vi "Values String Changed.vi"(8 "error in (no error)":errorcluster, 11 "Application Data in":T1 {"current buffer data"."channels"."configuration"."string offset" format="%d bytes"; "current buffer data"."avg bandwidth" format="%.0g bytes"}) -> (0 "error out":errorcluster, 3 "Application Data out":T1 {"current buffer data"."channels"."configuration"."string offset" format="%d bytes"; "current buffer data"."avg bandwidth" format="%.0g bytes"})   [LabVIEW 2017, in "Data Viewer.lvlib"]
uses:
  Core/VIs/Data Viewer/Source/Data Viewer.lvlib
  Application Data.ctl
  <vilib>/NI/Memory Manager/Classes/Pointer/Pointer.lvclass
  VeriStand/Data Sharing Custom Device/Source/DSF Core.lvlibp/Classes/Configuration/Core/Framework/Framework Configuration.lvclass
  Buffer Reader/Queue Data.ctl
  Buffer Reader/Buffer Data.ctl
  VeriStand/Data Sharing Custom Device/Source/DSF Core.lvlibp/Classes/Configuration/Core/Transfer/Channel Configuration.ctl
  VeriStand/Data Sharing Custom Device/Source/DSF Core.lvlibp/Typedefs/Core Channel Configuration.ctl
  VeriStand/Data Sharing Custom Device/Source/DSF Core.lvlibp/Typedefs/DSF Data Type.ctl
  VeriStand/Data Sharing Custom Device/Source/DSF Core.lvlibp/Typedefs/DSF Settings Info.ctl
  VeriStand/Data Sharing Custom Device/Source/DSF Core.lvlibp/Typedefs/DSF Byte Order.ctl
  VeriStand/Data Sharing Custom Device/Source/DSF Core.lvlibp/Classes/Thread/Data Server/DSF Buffer Subset Descriptor.ctl
  VeriStand/Data Sharing Custom Device/Source/DSF Core.lvlibp/Typedefs/DSF Buffer Type.ctl
  Values Channels.ctl
  VeriStand/Data Sharing Custom Device/Source/DSF Core.lvlibp/Classes/Framework/Framework.lvclass
  VeriStand/Data Sharing Custom Device/Source/DSF Core.lvlibp
  VeriStand/Data Sharing Custom Device/Source/DSF Core.lvlibp/Classes/Configuration/Core/Channel/Channel Configuration.lvclass
  VeriStand/Data Sharing Custom Device/Source/DSF Core.lvlibp/Classes/Configuration/Core/Transfer/Transfer Configuration.lvclass
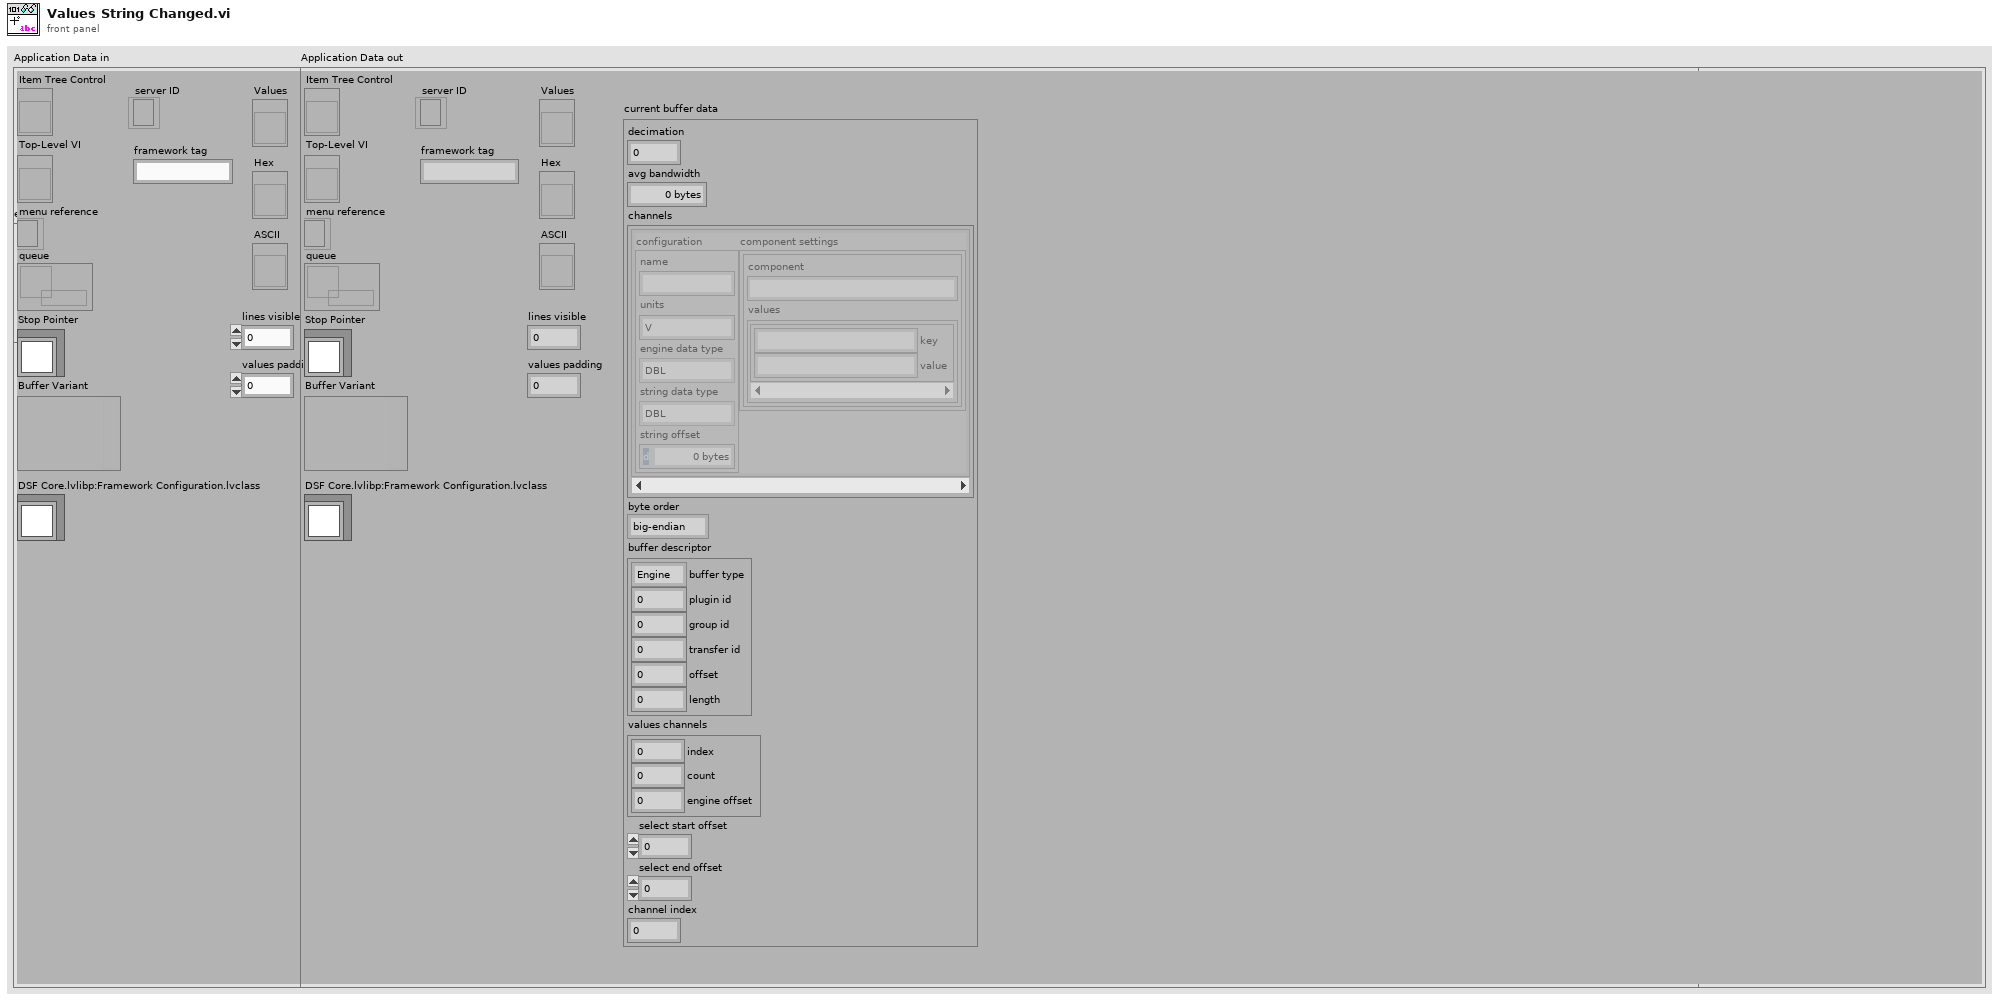
[diagram p1: front panel]
types:
  T1 = typedef "Data Viewer.lvlib/Application Data.ctl" = cluster{"Item Tree Control":refnum<vi>, "Top-Level VI":refnum<vi>, "menu reference":refnum<k9>, "queue":refnum<queue>, "Stop Pointer":refnum<class "Pointer.lvclass">, "Buffer Variant":variant, "server ID":refnum<k5>, "framework tag":string, "Values":refnum<vi>, "Hex":refnum<vi>, "ASCII":refnum<vi>, "lines visible":i32, "values padding":i32, "current buffer data":T2, "DSF Core.lvlibp:Framework Configuration.lvclass":refnum<class "Framework Configuration.lvclass">}
  T2 = typedef "Data Viewer.lvlib/Buffer Data.ctl" = cluster{"decimation":u64, "avg bandwidth":dbl, "channels":T3[], "byte order":T7, "buffer descriptor":T8, "values channels":T10, "select start offset":u64, "select end offset":u64, "channel index":i32}
  T3 = typedef "DSF Core.lvlibp/Transfer Configuration.lvclass/Channel Configuration.ctl" = cluster{"configuration":T4, "component settings":T6[]}
  T4 = typedef "DSF Core.lvlibp/Channel Configuration.lvclass/Core Channel Configuration.ctl" = cluster{"name":string, "units":string, "engine data type":T5, "string data type":T5, "string offset":u64}
  T5 = typedef "DSF Core.lvlibp/DSF Data Type.ctl" = enum8{"Bool", "SGL", "DBL", "I8", "I16", "I32", "I64", "U8", "U16", "U32", "U64"}
  T6 = typedef "DSF Core.lvlibp/DSF Settings Info.ctl" = cluster{"component":string, "values":cluster{"key":string, "value":string}[]}
  T7 = typedef "DSF Core.lvlibp/DSF Byte Order.ctl" = enum8{"big-endian", "little-endian"}
  T8 = typedef "DSF Core.lvlibp/DSF Buffer Subset Descriptor.ctl" = cluster{"buffer type":T9, "plugin id":i32, "group id":i32, "transfer id":i32, "offset":u64, "length":i64}
  T9 = typedef "DSF Core.lvlibp/DSF Buffer Type.ctl" = enum16{"Engine", "String"}
  T10 = typedef "Data Viewer.lvlib/Values Channels.ctl" = cluster{"index":i32, "count":i32, "engine offset":u64}
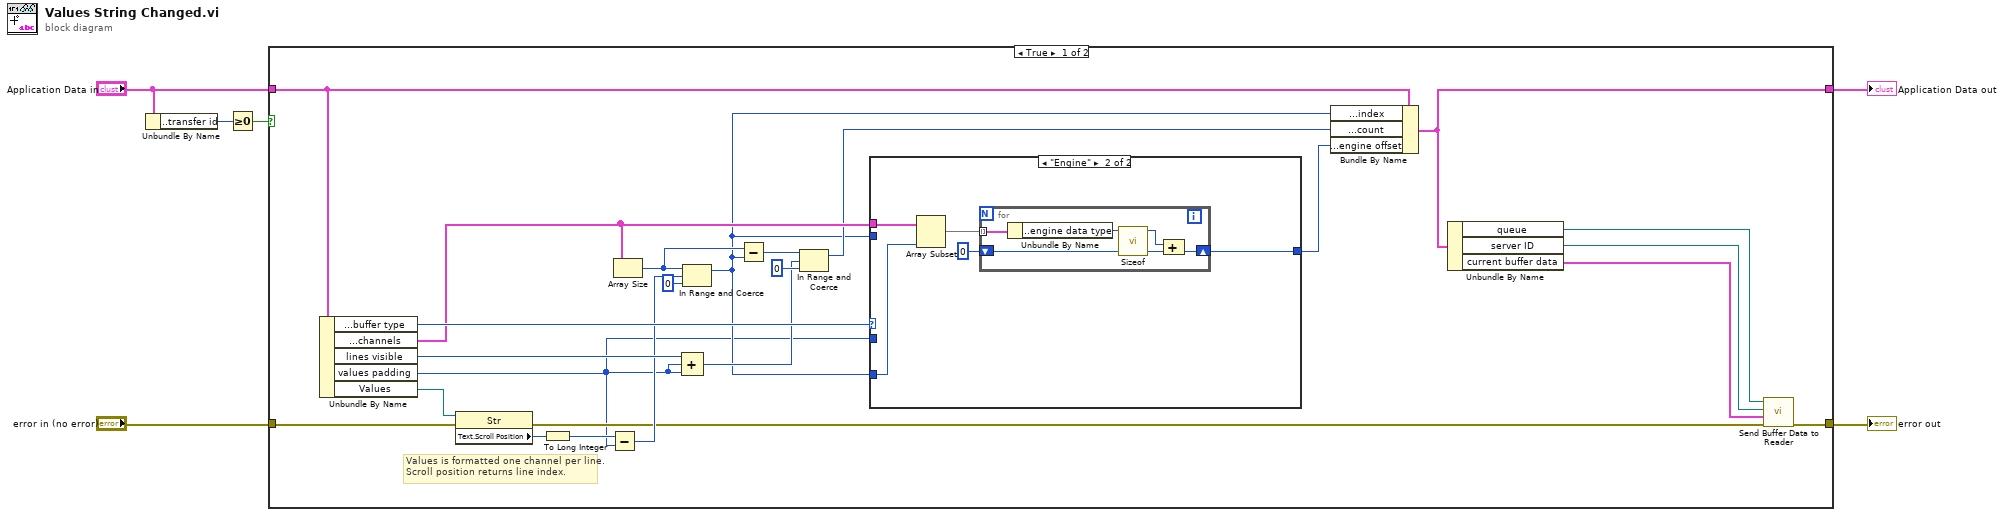
[diagram p0: block diagram]
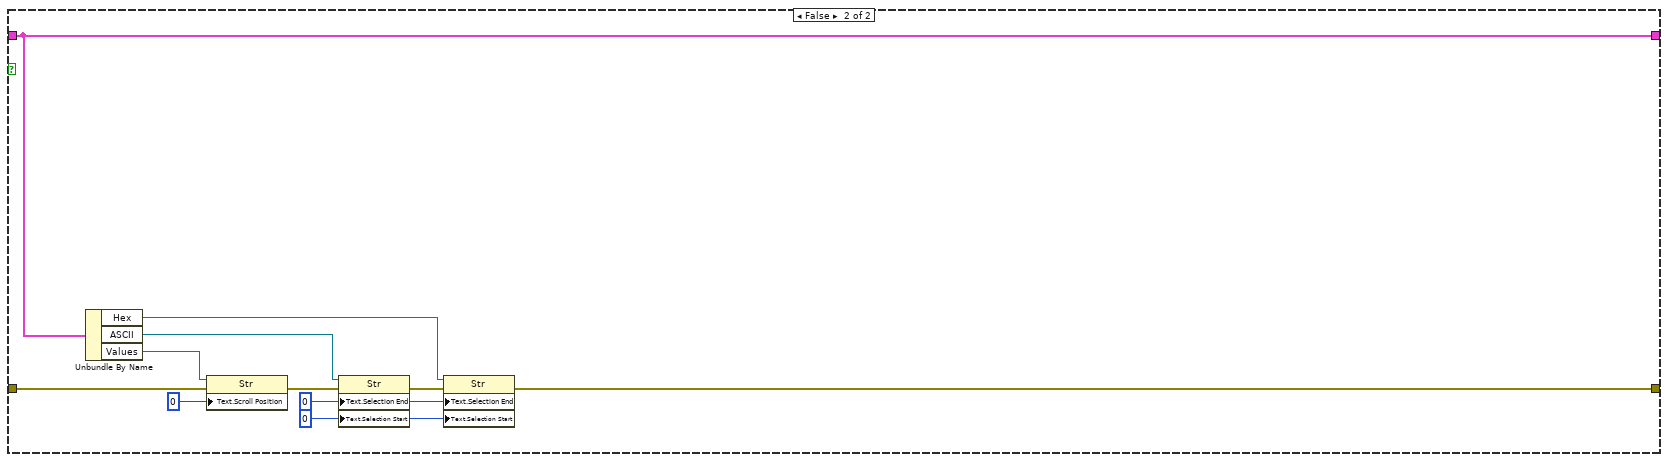
[diagram p3: hidden frame]
diagram:
  n1 = Unbundle By Name("Application Data in") -> ("current buffer data.buffer descriptor.transfer id"=w1:i32)
  n2 = Greater Or Equal To 0?(x=w1) -> (x >= 0?=w2:bool)
  n3 = case shown="True" w2 {
    tunnel: "error in (no error)" -> [w30 w50]
    tunnel: [w22 w47] -> w4
    tunnel: "Application Data in" -> [w25 w49]
    tunnel: [w18 w49] -> w5
    frame True {
      # "Values is formatted one channel per line. Scroll position returns line index."
      n4 = Unbundle By Name(w25) -> ("current buffer data.buffer descriptor.buffer type"=w24:T9, "current buffer data.channels"=w23:T3[], "lines visible"=w16:i32, "values padding"=w7:i32, "Values"=w26:refnum<vi>)
      n5 = property class="Str"(reference=w26, error in=w30) -> (error out=w8:errorcluster, "Text.Scroll Position"=w28:u32)  [unwired: 1 out]
      n6 = To Long Integer(number=w28) -> (32bit integer=w27:i32)
      n7 = Subtract(x=w27, y=w7) -> (x-y=w15:i32)
      n8 = Array Size(array=w23) -> (size(s)=w14:i32)
      n9 = Compound Arithmetic op=ADD(w16, w7, w7) -> (w10:i32)
      n10 = In Range and Coerce(upper limit=w14, x=w15, lower limit=0) -> (coerced(x)=w9:i32)  [unwired: 1 out]
      n11 = Subtract(x=w14, y=w9) -> (x-y=w12:i32)
      n12 = In Range and Coerce(upper limit=w12, x=w10, lower limit=0) -> (coerced(x)=w11:i32)  [unwired: 1 out]
      n13 = case shown="\"Engine\"" w24 {
        tunnel: w23 -> [_ w33]
        tunnel: w9 -> [_ _]
        tunnel: w9 -> [_ w32]
        tunnel: [_ w31] -> w17
        tunnel: w7 -> [_ _]
        frame "String" {
        }
        frame "Engine" {
          n14 = Array Subset(array=w33, length=w32) -> (w34:T3[])  [unwired: 1 in]
          n15 = for {
            tunnel: w34 -> [w40] mode=indexing
            shift-right: [w37] -> w31
            shift-left: u64 0 ("value") -> [w38]
            n16 = Unbundle By Name(w40) -> ("configuration.engine data type"=w39:T5)
            n17 = call "Sizeof.vi"("data type"=w39) -> ("size in bytes"=w36:u64)  [unwired: 9 in, 1 out]
            n18 = Compound Arithmetic op=ADD(w36, w38) -> (w37:u64)
          }
        }
      }
      n19 = Bundle By Name(cluster=w25, "current buffer data.values channels.index"=w9, "current buffer data.values channels.count"=w11, "current buffer data.values channels.engine offset"=w17) -> (w18:T1)
      n20 = Unbundle By Name(w18) -> ("queue"=w19:refnum<queue>, "server ID"=w20:refnum<k5>, "current buffer data"=w21:T2)
      n21 = call "Send Buffer Data to Reader.vi"("error in (no error)"=w8, "Buffer data"=w21, "server ID"=w20, "queue"=w19) -> ("error out"=w22:errorcluster)  [unwired: 7 in]
    }
    frame False {
      w42 = u32 0 ("Text.Selection:Start")
      w41 = u32 0 ("Text.Selection:End")
      n22 = Unbundle By Name(w49) -> ("Hex"=w43:refnum<vi>, "ASCII"=w44:refnum<vi>, "Values"=w46:refnum<vi>)
      n23 = property class="Str"(reference=w46, error in=w50, "Text.Scroll Position"=u32 0) -> (error out=w51:errorcluster)  [unwired: 1 out]
      n24 = property class="Str"(reference=w44, error in=w51, "Text.Selection End"=w41, "Text.Selection Start"=w42) -> (error out=w48:errorcluster)  [unwired: 1 out]
      n25 = property class="Str"(reference=w43, error in=w48, "Text.Selection End"=w41, "Text.Selection Start"=w42) -> (error out=w47:errorcluster)  [unwired: 1 out]
    }
  }
  "error out" <- w4
  "Application Data out" <- w5
